vi "Read Drive Train Status Ref.vi"(8 "error in (no error)":errorcluster, 11 "Drive Train in":refnum<class "Drive Train.lvclass">) -> (0 "error out":errorcluster, 2 "Drive Train Status Ref":refnum<vi>, 3 "Drive Train out":refnum<class "Drive Train.lvclass">)   [LabVIEW 2013, in "Logical Systems.lvlib" / "Drive Train.lvlib" / "Drive Train.lvclass"]
uses:
  Drive Train.lvclass
  Drive Train Status.ctl
  Drive Train.lvclass/Drive Train.ctl
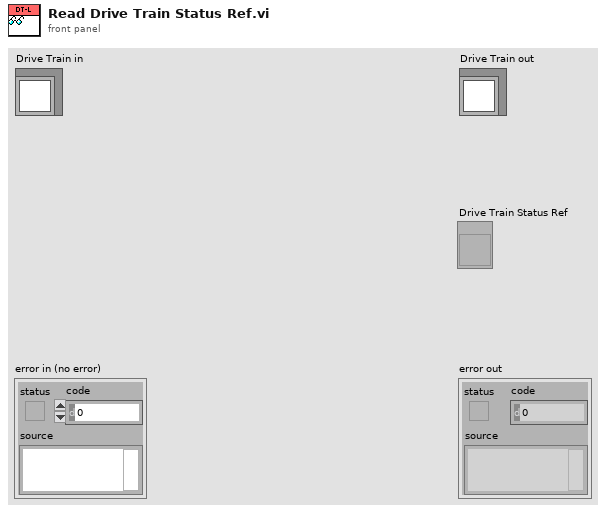
[diagram p1: front panel]
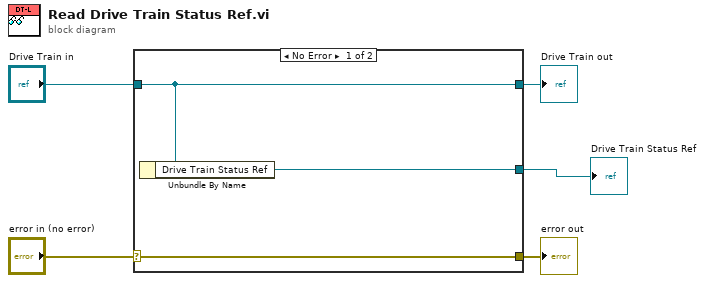
[diagram p0: block diagram]
diagram:
  n1 = case shown="No Error" "error in (no error)" {
    selector: "error in (no error)" -> [w8 w9]
    tunnel: [w8 w9] -> w4
    tunnel: [w7 w10] -> w2
    tunnel: "Drive Train in" -> [w7 w10]
    tunnel: [w6 _] -> w1
    frame No Error {
      n2 = Unbundle By Name(w7) -> ("Drive Train Status Ref"=w6:refnum<vi>)
    }
    frame Error {
    }
  }
  "error out" <- w4
  "Drive Train out" <- w2
  "Drive Train Status Ref" <- w1
